vi "Prefix Name.vi"(10 "Name":string, 11 "Prefix":T1) -> (2 "Prefixed Name":string)   [LabVIEW 2020, in "HTTP Utils.lvlib" / "Cookie.lvclass"]
uses:
  Cookie.lvclass
  Cookie Prefix.ctl
  HTTP Utils.lvlib
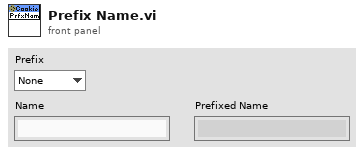
[diagram p1: front panel]
types:
  T1 = typedef "HTTP Utils.lvlib/Cookie Prefix.ctl" = enum16{"None", "Host", "Secure"}
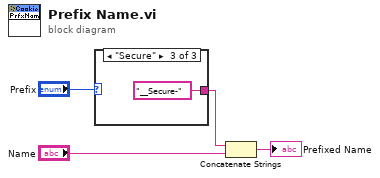
[diagram p0: block diagram]
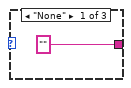
[diagram p2: hidden frame]
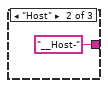
[diagram p3: hidden frame]
diagram:
  n1 = case shown="\"Secure\"" "Prefix" {
    tunnel: ["" "__Host-" "__Secure-"] -> w2
    frame "None" {
    }
    frame "Host" {
    }
    frame "Secure" {
    }
  }
  n2 = Concatenate Strings(w2, "Name") -> (→"Prefixed Name":string)
